vi "I2C NAU7802 Strain 24 Bit Gauge.vi"() -> ()   [LabVIEW 2020, in "CTI-Scratchpad.lvlib"]
uses:
  CTI-Scratchpad.lvlib
  CTI/Identity.ctl
  CTI-Peripheral/Analog Input/Adafruit I2C Strain Gauge/Private/NAU7802DataRate.ctl
  CTI-Peripheral/Analog Input/Adafruit I2C Strain Gauge/Private/NAU7802LDOVoltage.ctl
  CTI-Peripheral/Analog Input/Adafruit I2C Strain Gauge/Private/NAU7802PGA.ctl
  CTI-Peripheral/Analog Input/Adafruit I2C Strain Gauge/Private/ConfigDataCTRL0.ctl
  CTI/Error Reporting.ctl
  CTI-Peripheral/Analog Input/Adafruit I2C Strain Gauge/Private/ConfigDataCTRL1.ctl
  CTI/GPIO Number.ctl
  CTI/I2C Number.ctl
  CTI/Session/Session.lvclass
  CTI-Peripheral/Analog Input/Adafruit I2C Strain Gauge/Adafruit NAU7802 24bit Strain Gauge.lvclass
  CTI/VisaComms/VisaComms.lvclass
  CTI/CTI.lvlib
panel:
  out "Configure NAU7802 CTRL0 2":T1={"Register reset"=FALSE, "Power Up Digital cct"=TRUE, "Power Up Analog cct"=TRUE, "Power Up Ready"=TRUE, "Cycle Start"=TRUE, "Cycle Ready"=TRUE, "System Clock Select (Int 0)"=FALSE, "AVVD Source Select (AVVD Pin Input 0)"=TRUE}
  in  "Configure NAU7802 CTRL0":T1
  in  "PGA":T2=enum."x32"
  in  "LDOVoltage":T3=enum."3.6"
  in  "Data Rate":T4
  out "Waveform Chart":dbl(graph)=12214.0
  out "loop":i32=217
  in  "stop":bool
  out "Identity":T5={"Vendor"="CTI", "Model"="RP2040-Visa", "Serial"="E6626005A7352C2B", "Version"="0.9.2.20250711T143316Z"}
  in  "Grove Connector":enum16{"I2C0", "I2C1"}(ring)
  out "error out":errorcluster
  in  "Port":refnum<visa-resource-name>="ASRL27::INSTR"
  # "https://www.nuvoton.com/export/resource-files/en-us--DS_NAU7802_DataSheet_EN_Rev2.4.pdf"
  # "https://github.com/adafruit/Adafruit_NAU7802"
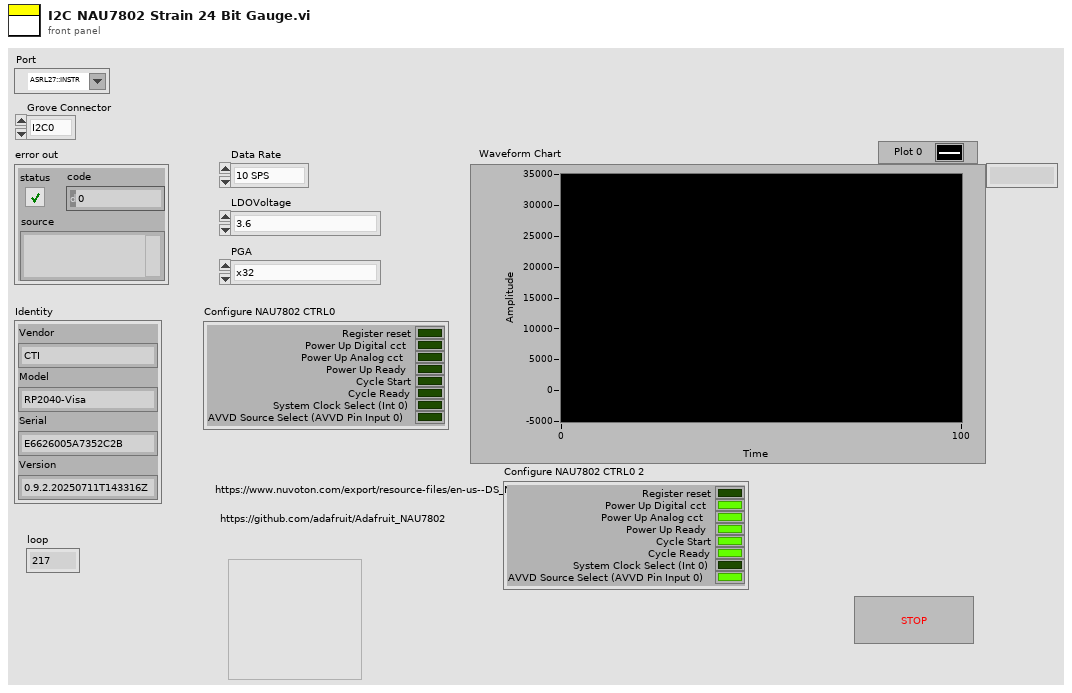
[diagram p1: front panel]
types:
  T1 = typedef "CTI-Peripheral.lvlib/Adafruit NAU7802 24bit Strain Gauge.lvclass/ConfigDataCTRL0.ctl" = cluster{"Register reset":bool, "Power Up Digital cct":bool, "Power Up Analog cct":bool, "Power Up Ready":bool, "Cycle Start":bool, "Cycle Ready":bool, "System Clock Select (Int 0)":bool, "AVVD Source Select (AVVD Pin Input 0)":bool}
  T2 = typedef "CTI-Peripheral.lvlib/Adafruit NAU7802 24bit Strain Gauge.lvclass/NAU7802PGA.ctl" = enum16{"x1", "x2", "x4", "x8", "x16", "x32", "x64", "x128"}
  T3 = typedef "CTI-Peripheral.lvlib/Adafruit NAU7802 24bit Strain Gauge.lvclass/NAU7802LDOVoltage.ctl" = enum16{"2.4", "2.7", "3.0", "3.3", "3.6", "3.9", "4.2", "4.5"}
  T4 = typedef "CTI-Peripheral.lvlib/Adafruit NAU7802 24bit Strain Gauge.lvclass/NAU7802DataRate.ctl" = enum16{"10 SPS", "20 SPS", "40 SPS", "80 SPS", "320 SPS"}
  T5 = typedef "CTI.lvlib/Identity.ctl" = cluster{"Vendor":string, "Model":string, "Serial":string, "Version":string}
  T6 = typedef "CTI-Peripheral.lvlib/Adafruit NAU7802 24bit Strain Gauge.lvclass/ConfigDataCTRL1.ctl" = cluster{"PGA":T2, "LDOVoltage":T3}
  T7 = typedef "CTI.lvlib/Error Reporting.ctl" = enum16{"Minimal", "Moderate", "Full"}
  T8 = typedef "CTI.lvlib/I2C Number.ctl" = i8
  T9 = typedef "CTI.lvlib/GPIO Number.ctl" = i8
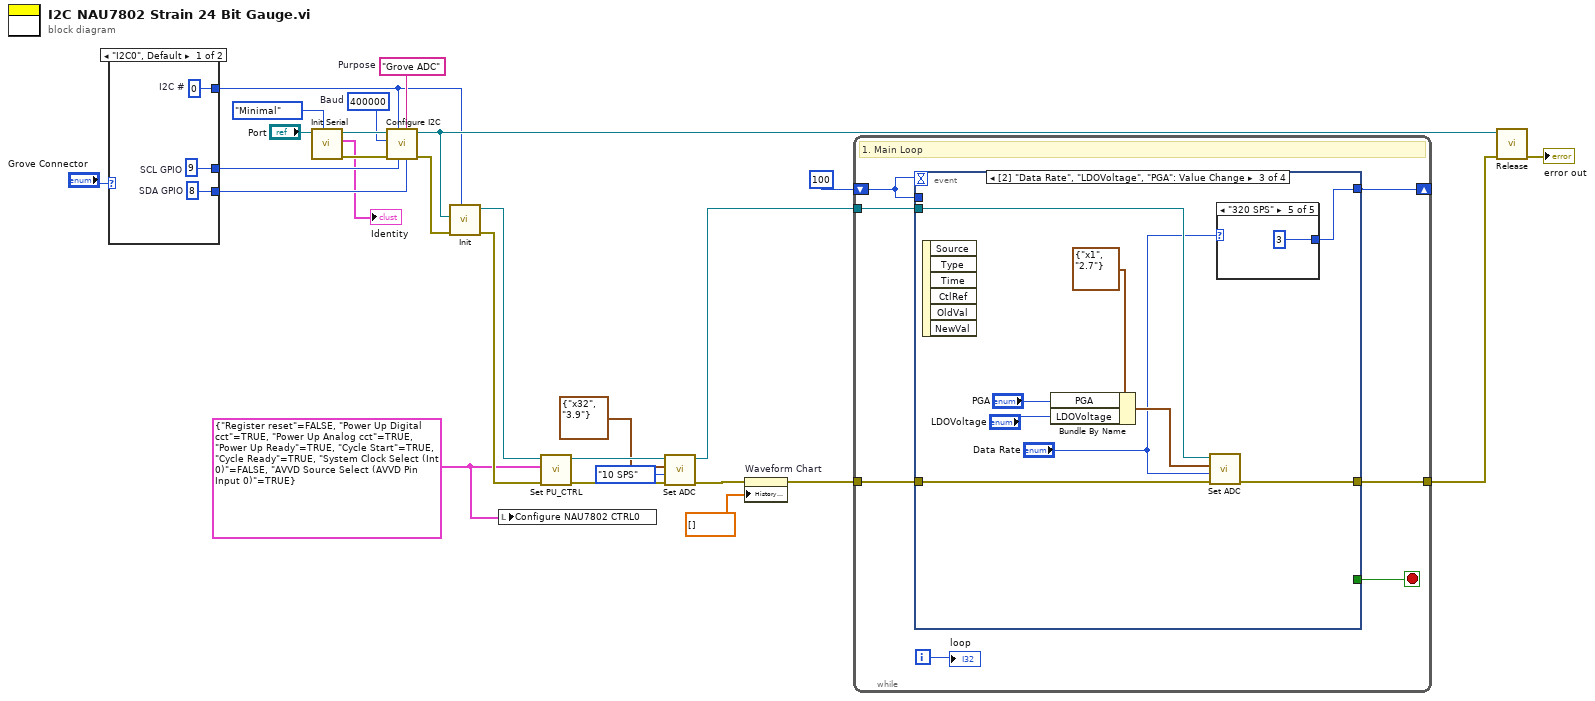
[diagram p0: block diagram]
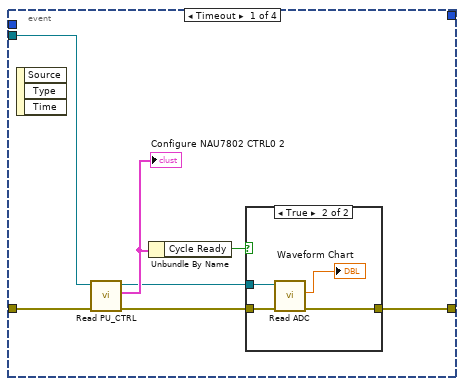
[diagram p2: hidden frame]
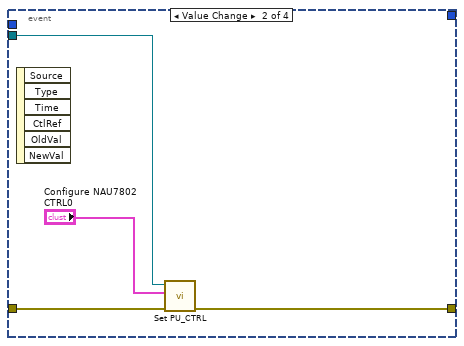
[diagram p4: hidden frame]
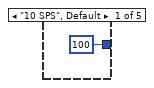
[diagram p5: hidden frame]
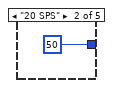
[diagram p6: hidden frame]
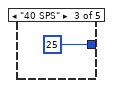
[diagram p7: hidden frame]
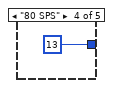
[diagram p8: hidden frame]
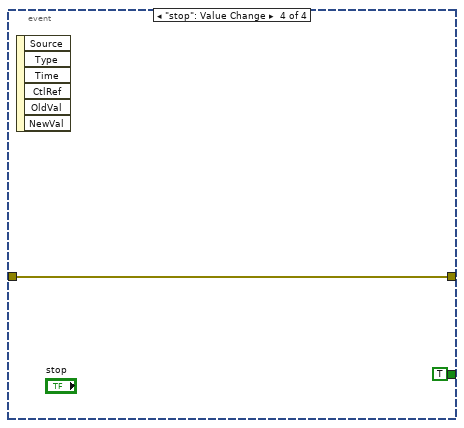
[diagram p9: hidden frame]
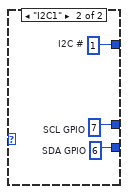
[diagram p10: hidden frame]
diagram:
  w2 = T1 {"Register reset"=FALSE, "Power Up Digital cct"=TRUE, "Power Up Analog cct"=TRUE, "Power Up Ready"=TRUE, "Cycle Start"=TRUE, "Cycle Ready"=TRUE, "System Clock Select (Int 0)"=FALSE, "AVVD Source Select (AVVD Pin Input 0)"=TRUE} ("Configure NAU7802 CTRL0")
  w22 = "Grove ADC"  # Purpose
  w23 = u32 400000  # Baud
  n1 = case shown="\"I2C0\", Default" "Grove Connector" {
    tunnel: [w30 w33] -> w18
    tunnel: [w29 w32] -> w17
    tunnel: [w28 w31] -> w16
    frame "I2C0", Default {
      w28 = T8 0  # I2C #
      w29 = T9 8  # SDA GPIO
      w30 = T9 9  # SCL GPIO
    }
    frame "I2C1" {
      w31 = T8 1  # I2C #
      w32 = T9 6  # SDA GPIO
      w33 = T9 7  # SCL GPIO
    }
  }
  n2 = call "Init Serial.vi"("Error Checking (Full)"=Error_Reporting."Minimal", "VISA resource name in"="Port") -> ("error out"=w24:errorcluster, "Identity"=→"Identity":T5, "Session"=w25:refnum<class "Session.lvclass">)  [unwired: 7 in]
  n3 = call "Configure I2C.vi"("SDA GPIO"=w17, "Purpose (\"I2C\")"=w22, "SCL GPIO"=w18, "I2C #"=w16, "error in (no error)"=w24, "Baud"=w23, "Session in"=w25) -> ("error out"=w21:errorcluster, "Session out"=w20:refnum<class "Session.lvclass">)  [unwired: 3 in]
  n4 = call "Init.vi"("I2C #"=w16, "error in (no error)"=w21, "Session In"=w20) -> ("error out"=w8:errorcluster, "NAU7802 Out"=w7:refnum<class "Adafruit NAU7802 24bit Strain Gauge.lvclass">)  [unwired: 7 in]
  n5 = local write "Configure NAU7802 CTRL0"(w2) -> ()
  n6 = call-dynamic "Set PU_CTRL.vi"("error in (no error)"=w8, "Configure NAU7802 CTRL0"=w2, "NAU7802 in"=w7) -> ("error out"=w5:errorcluster, "NAU7802 out"=w6:refnum<class "Adafruit NAU7802 24bit Strain Gauge.lvclass">)  [unwired: 7 in]
  n7 = call-dynamic "Set ADC.vi"("error in (no error)"=w5, "Data Rate"=NAU7802DataRate."10 SPS", "Configure NAU7802 CTRL1"=T6 {"PGA"=enum."x32", "LDOVoltage"=enum."3.9"}, "NAU7802 in"=w6) -> ("error out"=w9:errorcluster, "NAU7802 out"=w10:refnum<class "Adafruit NAU7802 24bit Strain Gauge.lvclass">)  [unwired: 6 in]
  n8 = property on="Waveform Chart" class="WFChart (strict)"(error in=w9, "History Data"=dbl[] []) -> (error out=w11:errorcluster)  [unwired: 1 in, 1 out]
  n9 = while {
    tunnel: w11 -> [w39]
    tunnel: w10 -> [w40]
    tunnel: [w37] -> w14
    shift-right: [w34] -> _
    shift-left: 100 -> [w35]
    i -> [w38]
    stop <- w36 stop-if-true
    # "1. Main Loop"
    n10 = event shown="[2] \"Data Rate\", \"LDOVoltage\", \"PGA\": Value Change" {
      selector: _ -> [_ _ _ _]
      dyn-events: _ -> [_ _ _ _]
      timeout: w35 -> [_ _ _ _]
      tunnel: w40 -> [w47 w53 w65 _]
      tunnel: w39 -> [w46 w55 w63 w71]
      tunnel: [w41 w54 w64 w71] -> w37
      tunnel: [_ _ _ TRUE] -> w36
      tunnel: w35 -> [_ _ _ _]
      tunnel: [_ _ w57 _] -> w34
      event Timeout {
        n11 = event-data() -> ()  [unwired: 1 in, 3 out]
        n12 = call-dynamic "Read PU_CTRL.vi"("error in (no error)"=w46, "NAU7802 in"=w47) -> ("error out"=w43:errorcluster, "Configure NAU7802 CTRL0"=w45:T1, "NAU7802 out"=w42:refnum<class "Adafruit NAU7802 24bit Strain Gauge.lvclass">)  [unwired: 7 in]
        "Configure NAU7802 CTRL0 2" <- w45
        n13 = Unbundle By Name(w45) -> ("Cycle Ready"=w44:bool)
        n14 = case shown="True" w44 {
          tunnel: w43 -> [w48 w51]
          tunnel: w42 -> [_ w52]
          tunnel: [w48 w49] -> w41
          frame False {
          }
          frame True {
            n15 = call-dynamic "Read ADC.vi"("error in (no error)"=w51, "NAU7802 in"=w52) -> ("error out"=w49:errorcluster, "Data Out"=→"Waveform Chart":dbl)  [unwired: 7 in, 1 out]
          }
        }
      }
      event Value Change {
        n16 = event-data() -> ()  [unwired: 1 in, 6 out]
        n17 = call-dynamic "Set PU_CTRL.vi"("error in (no error)"=w55, "Configure NAU7802 CTRL0"="Configure NAU7802 CTRL0", "NAU7802 in"=w53) -> ("error out"=w54:errorcluster)  [unwired: 7 in, 1 out]
      }
      event Value Change {
        n18 = event-data() -> ()  [unwired: 1 in, 6 out]
        n19 = Bundle By Name(cluster=T6 {"PGA"=enum."x1", "LDOVoltage"=enum."2.7"} ("Configure NAU7802 CTRL1"), "PGA"="PGA", "LDOVoltage"="LDOVoltage") -> (w62:T6)
        n20 = call-dynamic "Set ADC.vi"("error in (no error)"=w63, "Data Rate"="Data Rate", "Configure NAU7802 CTRL1"=w62, "NAU7802 in"=w65) -> ("error out"=w64:errorcluster)  [unwired: 6 in, 1 out]
        n21 = case shown="\"320 SPS\"" "Data Rate" {
          tunnel: [100 50 25 13 3] -> w57
          frame "10 SPS", Default {
          }
          frame "20 SPS" {
          }
          frame "40 SPS" {
          }
          frame "80 SPS" {
          }
          frame "320 SPS" {
          }
        }
      }
      event "stop": Value Change {
        n22 = event-data() -> ()  [unwired: 1 in, 6 out]
      }
    }
    "loop" <- w38
  }
  n23 = call-dynamic "Release.vi"("error in (no error)"=w14, "Session in"=w20) -> ("error out"=→"error out":errorcluster)  [unwired: 9 in]
